vi "Index_Sensors.vi"() -> (1 "Intake Pressed":bool, 2 "Reject Pressed":bool, 3 "Elevate Pressed":bool)   [LabVIEW 2020]
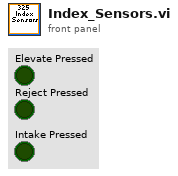
[diagram p1: front panel]
types:
  T1 = typedef "WPI_SwitchDevRef.ctl" = cluster{"DevStatus":errorcluster, "DIO Channel":T2, "CntIndex":T3, "Normally Closed":bool}
  T2 = typedef "FPGA_DIOChannel.ctl" = enum8{"DIO 0", "DIO 1", "DIO 2", "DIO 3", "DIO 4", "DIO 5", "DIO 6", "DIO 7", "DIO 8", "DIO 9", "DIO MXP 0", "DIO MXP 1", "DIO MXP 2", "DIO MXP 3", "DIO MXP 4", "DIO MXP 5", "DIO MXP 6", "DIO MXP 7", "DIO MXP 8", "DIO MXP 9", "DIO MXP 10", "DIO MXP 11", "DIO MXP 12", "DIO MXP 13", "DIO MXP 14", "DIO MXP 15", "SPI Port CS1", "SPI Port CS2", "SPI Port CS3", "SPI Port MISO", "SPI Port MOSI", "Invalid"}
  T3 = typedef "FPGA_CounterCtrSystemIndex.ctl" = enum8{"Ctr 0", "Ctr 1", "Ctr 2", "Ctr 3", "Ctr 4", "Ctr 5", "Ctr 6", "Ctr 7", "Invalid"}
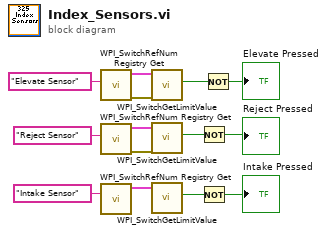
[diagram p0: block diagram]
diagram:
  n1 = call <vilib>:"WPI_SwitchRefNum Registry Get.vi"("refnum name"="Elevate Sensor") -> ("error out"=w9:errorcluster, "SwitchDevRef"=w8:T1)  [unwired: 9 in]
  n2 = call <vilib>:"WPI_SwitchRefNum Registry Get.vi"("refnum name"="Reject Sensor") -> ("error out"=w14:errorcluster, "SwitchDevRef"=w13:T1)  [unwired: 9 in]
  n3 = call <vilib>:"WPI_SwitchRefNum Registry Get.vi"("refnum name"="Intake Sensor") -> ("SwitchDevRef"=w10:T1)  [unwired: 9 in, 1 out]
  n4 = call <vilib>:"WPI_SwitchGetLimitValue.vi"("error in (no error)"=w9, "SwitchDevRef"=w8) -> ("Switch Pressed"=w6:bool)  [unwired: 7 in, 2 out]
  n5 = call <vilib>:"WPI_SwitchGetLimitValue.vi"("error in (no error)"=w14, "SwitchDevRef"=w13) -> ("Switch Pressed"=w4:bool)  [unwired: 7 in, 2 out]
  n6 = call <vilib>:"WPI_SwitchGetLimitValue.vi"("SwitchDevRef"=w10) -> ("Switch Pressed"=w2:bool)  [unwired: 8 in, 2 out]
  n7 = Not(x=w4) -> (.not. x?=→"Reject Pressed":bool)
  n8 = Not(x=w2) -> (.not. x?=→"Intake Pressed":bool)
  n9 = Not(x=w6) -> (.not. x?=→"Elevate Pressed":bool)
